vi "v4.1.vi"() -> ()   [LabVIEW 2018]
uses:
  <vilib>/DAQmx/read.llb/DAQmx Read (Analog 1D DBL NChan 1Samp).vi
  <extravilib>/ChannelInstances/High Speed Stream-c(a[.](c(dbl,dbl,dbl,dbl)),stamp,a[.](dbl),c(dbl,dbl,dbl,dbl,dbl,dbl,dbl))/_Read For Replicate.vi
  <extravilib>/ChannelInstances/High Speed Stream-c(a[.](c(dbl,dbl,dbl,dbl)),stamp,a[.](dbl),c(dbl,dbl,dbl,dbl,dbl,dbl,dbl))/Instantiate.vi
  <extravilib>/ChannelInstances/High Speed Stream-c(a[.](c(dbl,dbl,dbl,dbl)),stamp,a[.](dbl),c(dbl,dbl,dbl,dbl,dbl,dbl,dbl))/)Channel.vi
  <extravilib>/ChannelInstances/High Speed Stream-c(a[.](c(dbl,dbl,dbl,dbl)),stamp,a[.](dbl),c(dbl,dbl,dbl,dbl,dbl,dbl,dbl))/Abort Signal/Init Signal.vi
  <vilib>/Utility/file.llb/Write Delimited Spreadsheet (string).vi
  <vilib>/DAQmx/create/channels.llb/DAQmx Create Channel (AI-Temperature-Thermocouple).vi
  <vilib>/DAQmx/configure/timing.llb/DAQmx Timing (Sample Clock).vi
  <vilib>/DAQmx/miscellaneous.llb/DAQmx Fill In Error Info.vi
  <extravilib>/ChannelInstances/High Speed Stream-c(a[.](c(dbl,dbl,dbl,dbl)),stamp,a[.](dbl),c(dbl,dbl,dbl,dbl,dbl,dbl,dbl)).lvlib
  <resource>/objmgr/daqmx.rc
panel:
  out "Actual Sample Rate":dbl
  out "Export Timestamp":timestamp format="%<%H:%M:%S>T"
  out "Rig Temperatures":T1
  out "Flowrate Data":T2(array[cluster])
  out "UI Timestamp":timestamp format="%<%X\n%x>T"
  out "DAQ Timestamp":timestamp format="%<%H:%M:%S>T"
  in  "file path (dialog if empty)":path
  out "Enum":T3(ring)
  in  "Start Recording?":bool
  in  "Stop Recording?":bool
  in  "Flowrate Control":dbl
  out "Status":T4(ring)
  in  "OK Button":bool
  in  "DAQ Properties":cluster{"Sample Rate [Hz]":dbl}={"Sample Rate [Hz]"=1.0} {"Sample Rate [Hz]" min=0.1 max=10000.0 step=0.1}
  # "Line Data [ °C]"
  # "Rig Temperatures [ °C]"
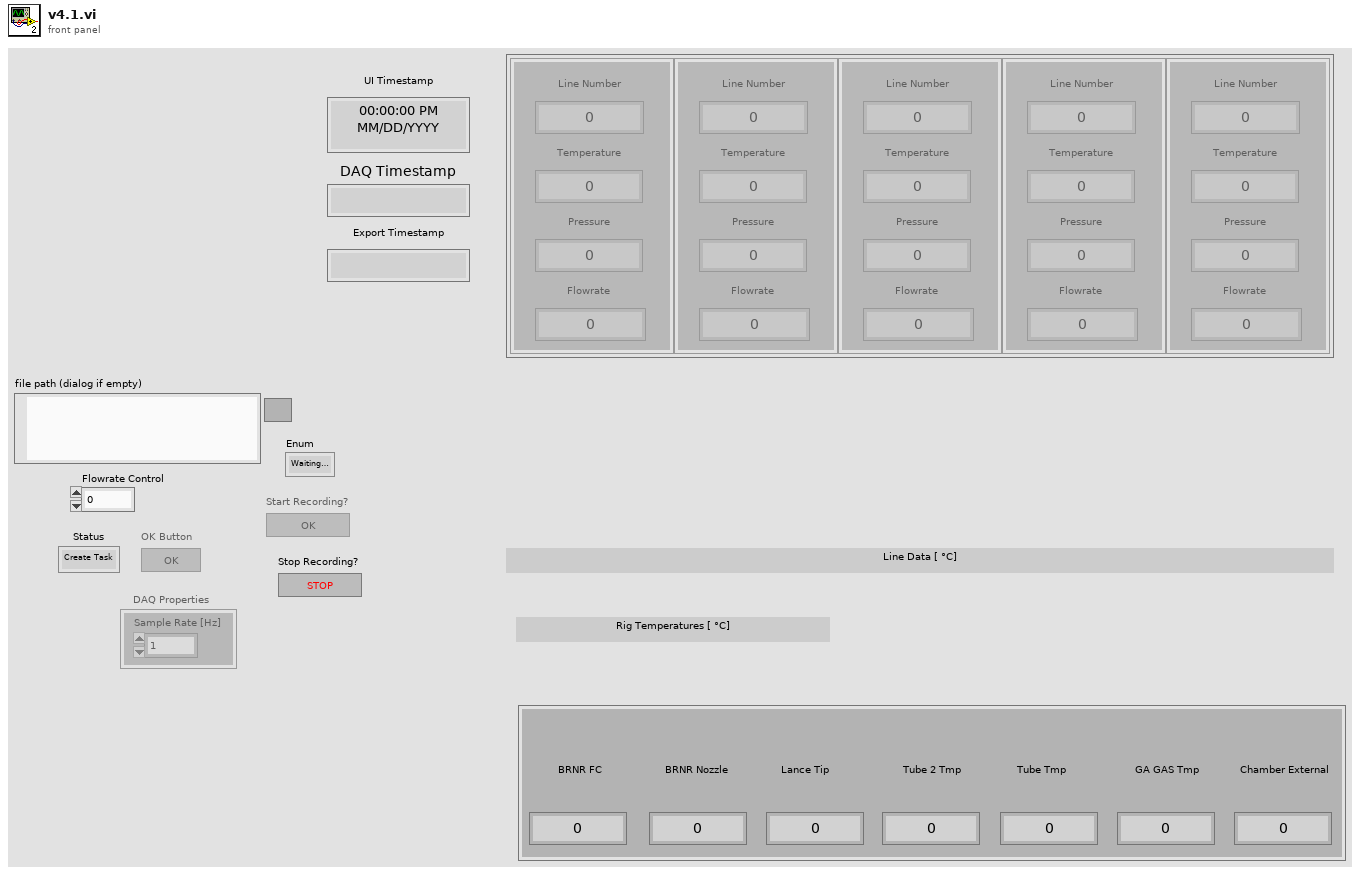
[diagram p1: front panel]
types:
  T1 = cluster{"BRNR FC":dbl, "BRNR Nozzle":dbl, "Lance Tip":dbl, "Tube 2 Tmp":dbl, "Tube Tmp":dbl, "GA GAS Tmp":dbl, "Chamber External":dbl}
  T2 = cluster{"Line Number":dbl, "Temperature":dbl, "Pressure":dbl, "Flowrate":dbl}[]
  T3 = enum16{"Waiting to record", "Creating Spreadsheet", "Recording", "Finished Recording"}
  T4 = enum16{"Create Task", "Change Settings", "Check Settings", "Read Data", "End Task"}
  T5 = enum8{"Enabled", "Disabled", "Disabled and Grayed Out"}
  T6 = cluster{"Flowrate Data":cluster{"Line Number":dbl, "Temperature":dbl, "Pressure":dbl, "Flowrate":dbl}[], "Current Time":timestamp, "DAQmx Data":dbl[], "Rig Temperatures":cluster{"BRNR FC":dbl, "BRNR Nozzle":dbl, "Lance Tip":dbl, "Tube 2 Tmp":dbl, "Tube Tmp":dbl, "GA GAS Tmp":dbl, "Chamber External Temp":dbl}}
  T7 = cluster{"BRNR FC":dbl, "BRNR Nozzle":dbl, "Lance Tip":dbl, "Tube 2 Tmp":dbl, "Tube Tmp":dbl, "GA GAS Tmp":dbl, "Chamber External Temp":dbl}
  T8 = typedef "High Speed Stream-c(a[.](c(dbl,dbl,dbl,dbl)),stamp,a[.](dbl),c(dbl,dbl,dbl,dbl,dbl,dbl,dbl)).lvlib/)Channel.ctl" = refnum<queue>
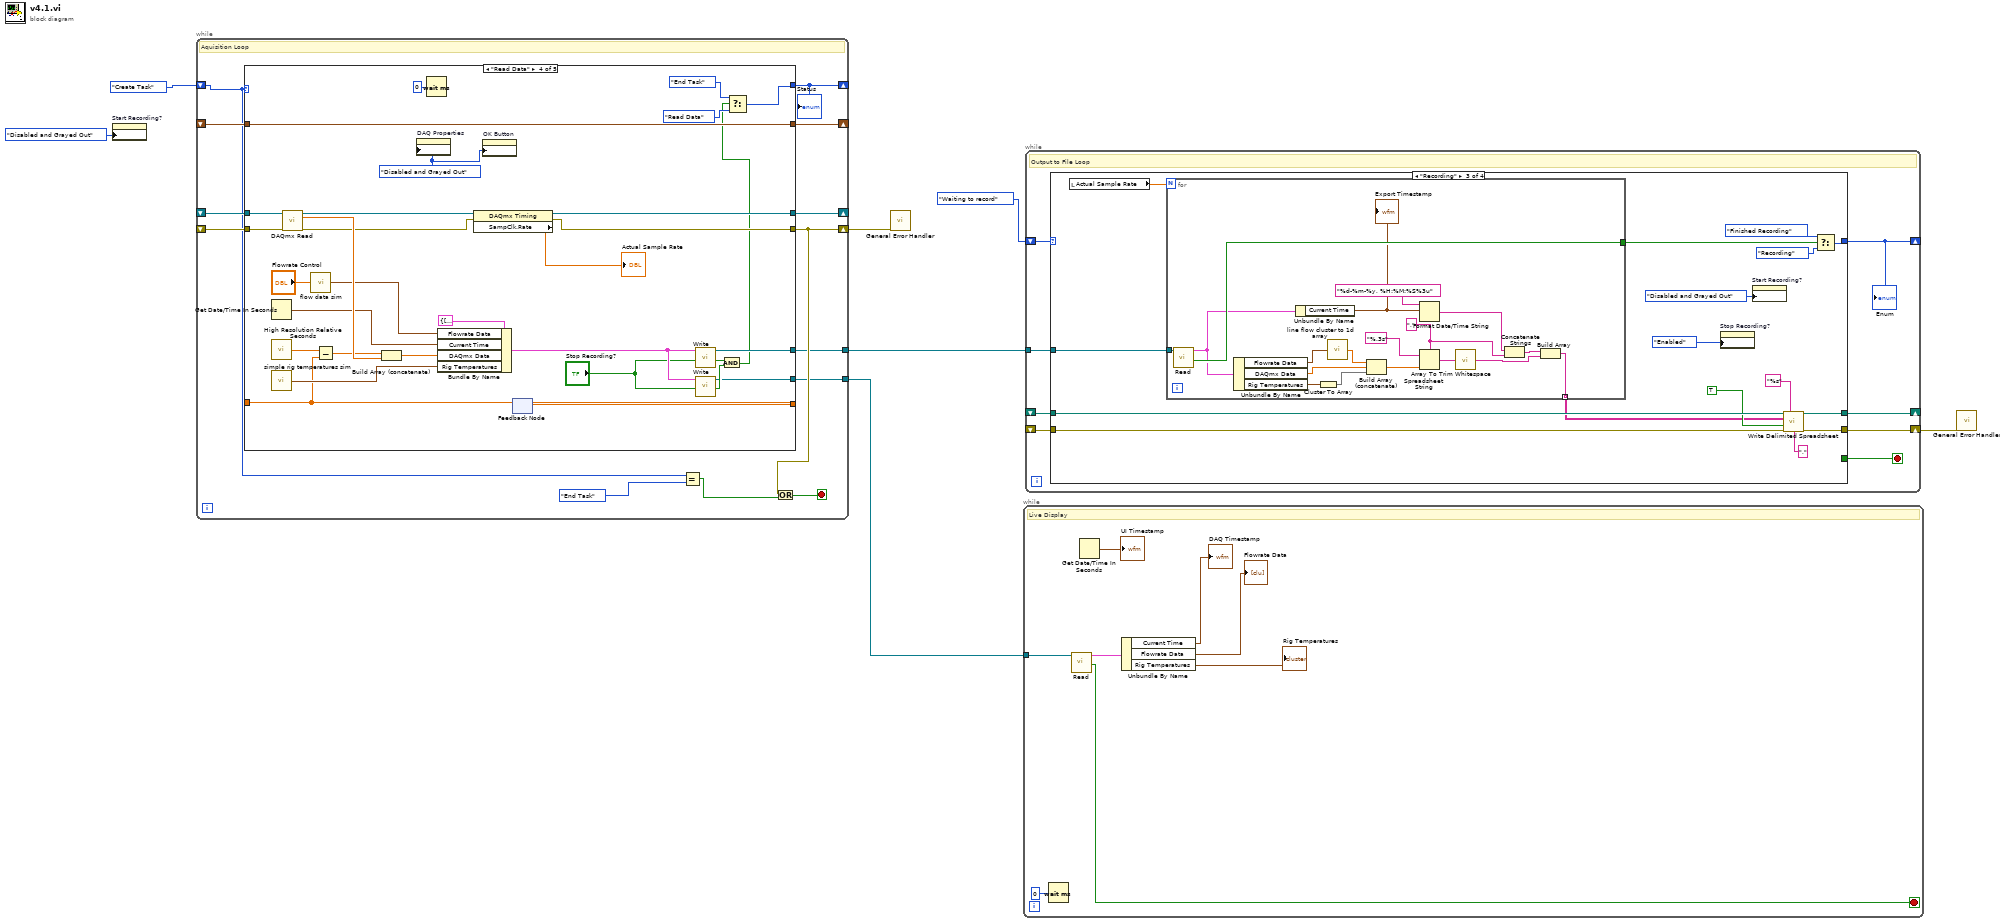
[diagram p0: block diagram]
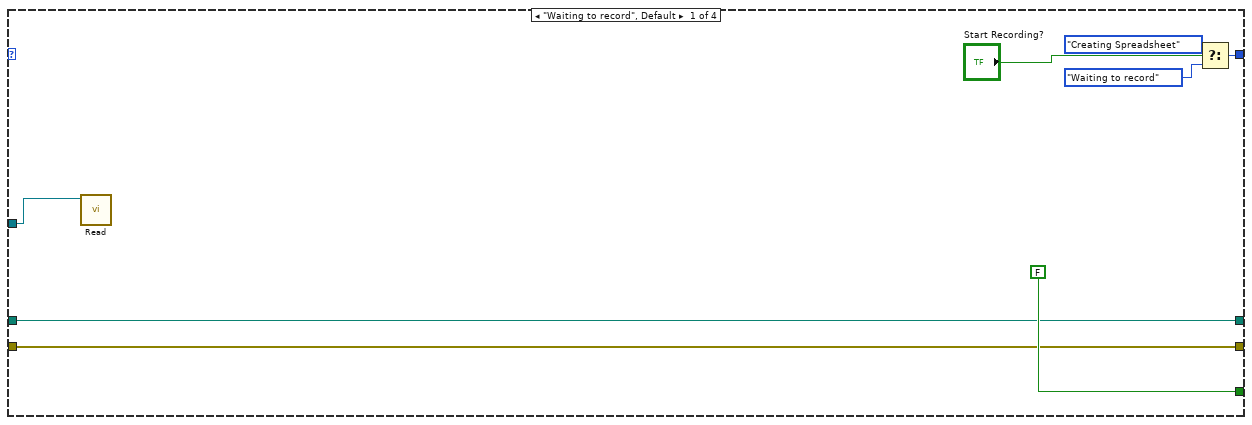
[diagram p2: hidden frame]
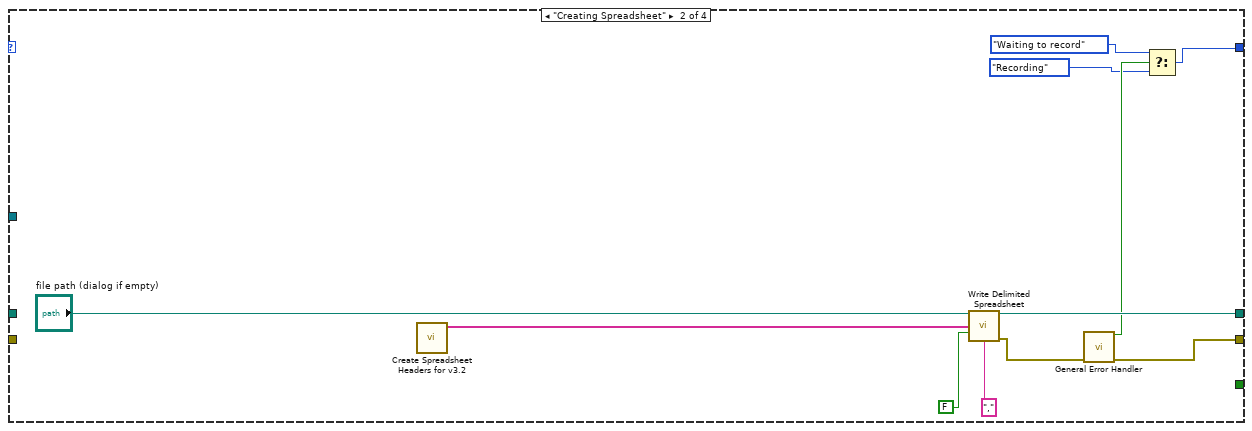
[diagram p3: hidden frame]
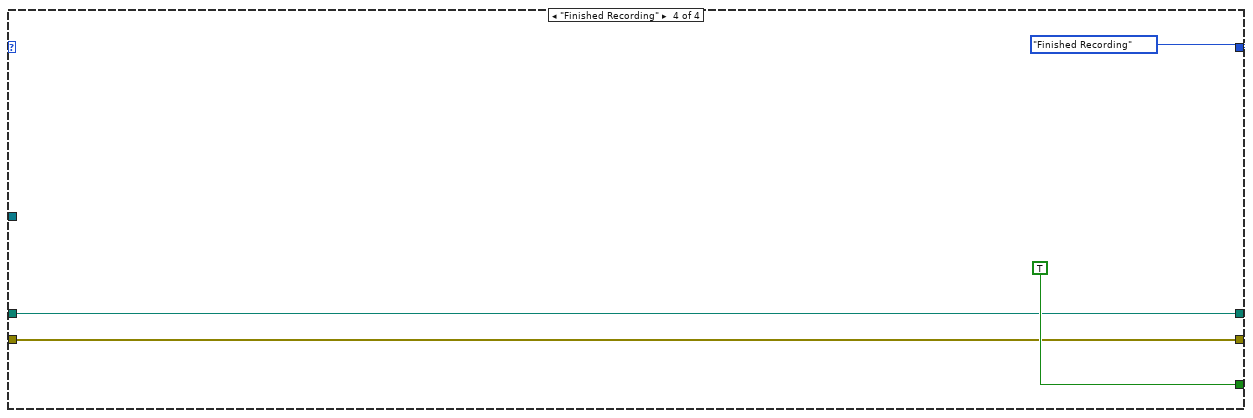
[diagram p4: hidden frame]
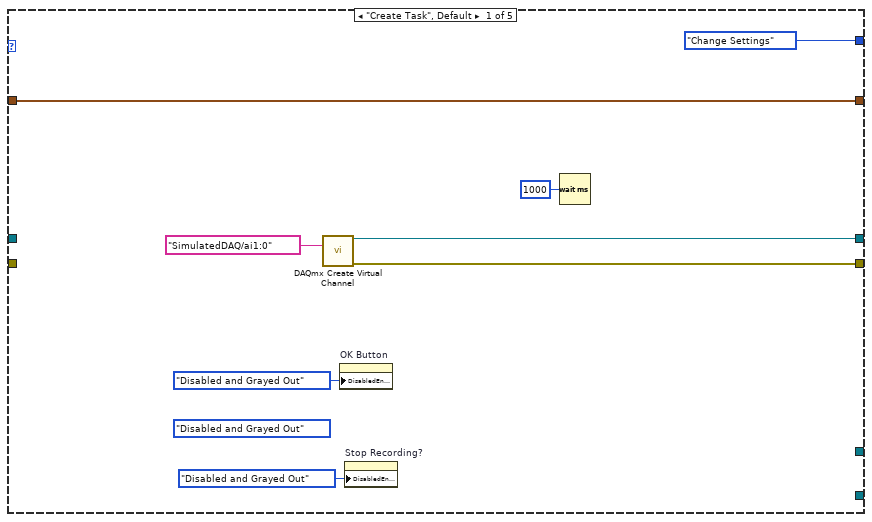
[diagram p5: hidden frame]
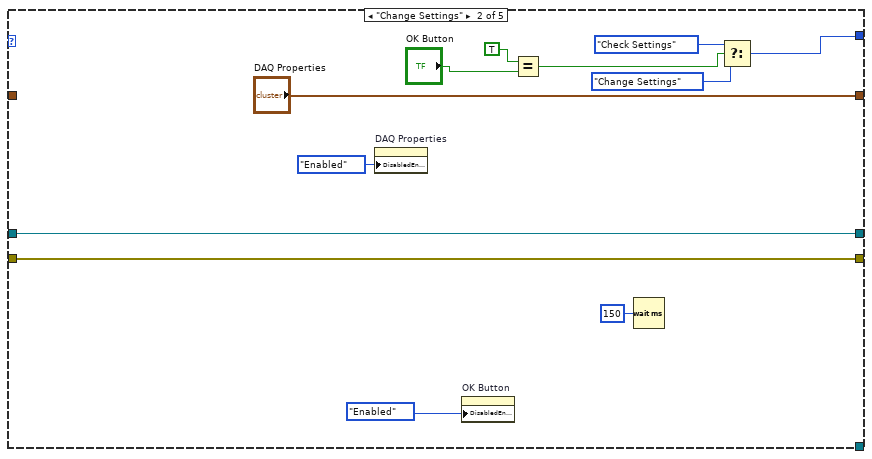
[diagram p6: hidden frame]
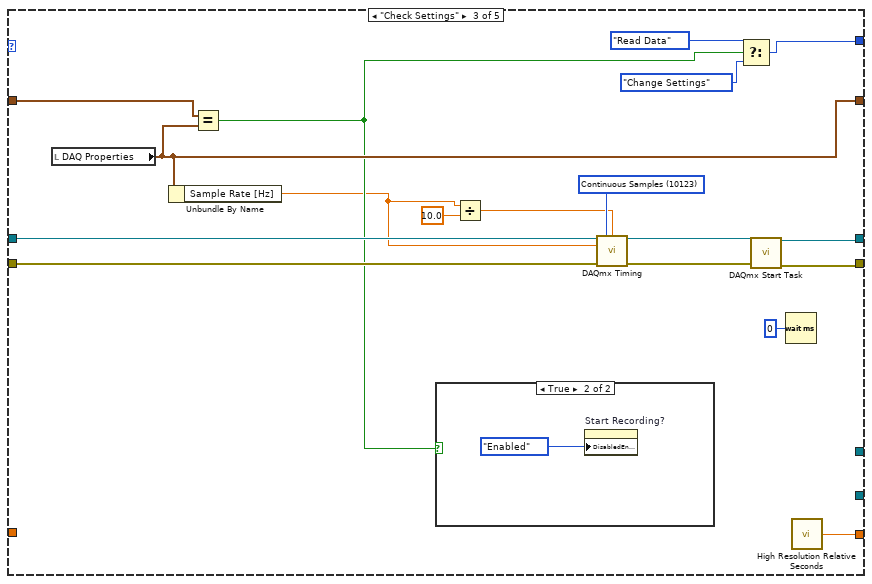
[diagram p7: hidden frame]
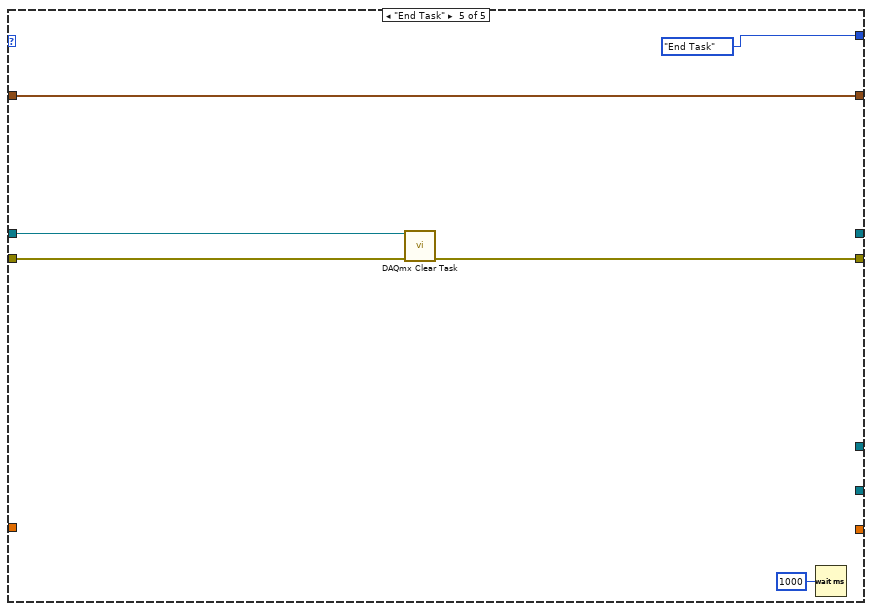
[diagram p9: hidden frame]
diagram:
  n1 = property on="Start Recording?" class="Bool"("DisabledEnum"=T5."Disabled and Grayed Out" ("Disabled")) -> ()  [unwired: 2 in, 2 out]
  n2 = while {
    shift-right: [w17] -> _
    shift-left: T4."Create Task" -> [w13]
    shift-right: [w22] -> _
    shift-left: _ -> [w20]
    shift-right: [w16] -> w3
    shift-left: _ -> [w19]
    shift-right: [w21] -> _
    shift-left: _ -> [w18]
    tunnel: [w11] -> w5
    tunnel: [w10] -> w1
    stop <- w12 stop-if-true
    # "Aquisition Loop"
    n3 = feedback #1() -> (w8:dbl)  [unwired: 1 in]
    n4 = case shown="\"Read Data\"" w13 {
      tunnel: [w30 w42 w50 w70 _] -> w22
      tunnel: [w29 w41 w49 w71 w97] -> w16
      tunnel: [T4."Change Settings" w35 w56 w87 T4."End Task"] -> w17
      tunnel: [w26 "DAQ Properties" w53 w89 w96] -> w21
      tunnel: w20 -> [_ w42 w55 w91 w94]
      tunnel: w19 -> [_ w41 w54 w90 w93]
      tunnel: w18 -> [w26 _ w60 w89 w96]
      tunnel: [_ _ _ w78 _] -> w11
      tunnel: [_ _ _ w67 _] -> w10
      tunnel: [_ _ w43 w62 _] -> w9
      tunnel: w8 -> [_ _ _ w62 _]
      frame "Create Task", Default {
        (unwired) T5."Disabled and Grayed Out" ("Disabled")
        n5 = call-poly <vilib>:"DAQmx Create Virtual Channel.vi"("physical channels"=tag "SimulatedDAQ/ai1:0") -> ("task out"=w30:refnum<k21>, "error out"=w29:errorcluster)  [unwired: 13 in]
        n6 = property on="OK Button" class="Bool"("DisabledEnum"=T5."Disabled and Grayed Out" ("Disabled")) -> ()  [unwired: 2 in, 2 out]
        n7 = property on="Stop Recording?" class="Bool"("DisabledEnum"=T5."Disabled and Grayed Out" ("Disabled")) -> ()  [unwired: 2 in, 2 out]
        n8 = Wait (ms)(milliseconds to wait=u32 1000) -> ()  [unwired: 1 out]
      }
      frame "Change Settings" {
        n9 = property on="DAQ Properties" class="Clust (strict)"("DisabledEnum"=T5."Enabled" ("Disabled")) -> ()  [unwired: 2 in, 2 out]
        n10 = property on="OK Button" class="Bool"("DisabledEnum"=T5."Enabled" ("Disabled")) -> ()  [unwired: 2 in, 2 out]
        n11 = Equal?(x=TRUE, y="OK Button") -> (x = y?=w37:bool)
        n12 = Wait (ms)(milliseconds to wait=u32 150) -> ()  [unwired: 1 out]
        n13 = Select(t=T4."Check Settings", s=w37, f=T4."Change Settings") -> (s? t:f=w35:T4)
      }
      frame "Check Settings" {
        w48 = 10123 items=["Finite Samples"=10178, "Continuous Samples"=10123, "Hardware Timed Single Point"=12522] ("sample mode")
        n14 = local read "DAQ Properties"() -> (w53:cluster{"Sample Rate [Hz]":dbl})
        n15 = Unbundle By Name(w53) -> ("Sample Rate [Hz]"=w45:dbl)
        n16 = Equal?(x=w60, y=w53) -> (x = y?=w47:bool)
        n17 = case shown="True" w47 {
          frame False {
          }
          frame True {
            n18 = property on="Start Recording?" class="Bool"("DisabledEnum"=T5."Enabled" ("Disabled")) -> ()  [unwired: 2 in, 2 out]
          }
        }
        n19 = Divide(x=w45, y=10.0) -> (x/y=w44:dbl)
        n20 = call-poly <vilib>:"DAQmx Timing.vi"("task/channels in"=w55, "sample mode"=w48, "samples per channel"=w44, "rate"=w45, "error in"=w54) -> ("task out"=w52:refnum<k21>, "error out"=w51:errorcluster)  [unwired: 9 in]
        n21 = Select(t=T4."Read Data", s=w47, f=T4."Change Settings") -> (s? t:f=w56:T4)
        n22 = call <vilib>:"DAQmx Start Task.vi"("task/channels in"=w52, "error in"=w51) -> ("task out"=w50:refnum<k21>, "error out"=w49:errorcluster)  [unwired: 12 in]
        n23 = Wait (ms)(milliseconds to wait=u32 0) -> ()  [unwired: 1 out]
        n24 = call <vilib>:"High Resolution Relative Seconds.vi"() -> ("relative seconds"=w43:dbl)
      }
      frame "Read Data" {
        w77 = T5."Disabled and Grayed Out" ("Disabled")
        n25 = Get Date/Time In Seconds() -> (seconds since 1Jan1904=w81:timestamp)
        n26 = call <vilib>:"High Resolution Relative Seconds.vi"() -> ("relative seconds"=w66:dbl)
        n27 = call "simple rig temperatures sim.vi"() -> ("Rig Temperatures"=w79:T7)
        n28 = call-poly <vilib>:"DAQmx Read.vi"("task/channels in"=w91, "error in"=w90) -> ("task out"=w72:refnum<k21>, "data"=w84:dbl[], "error out"=w69:errorcluster)  [unwired: 11 in]
        n29 = call "flow data sim.vi"("Offset"="Flowrate Control") -> ("Flowrate Data"=w80:T2)
        n30 = Subtract(x=w66, y=w62) -> (x-y=w63:dbl)
        n31 = Build Array (concatenate)(w63, w84) -> (w64:dbl[])
        n32 = property on="DAQ Properties" class="Clust (strict)"("DisabledEnum"=w77) -> ()  [unwired: 2 in, 2 out]
        n33 = Wait (ms)(milliseconds to wait=u32 0) -> ()  [unwired: 1 out]
        n34 = Bundle By Name(cluster=T6 {"Flowrate Data"=[{"Line Number"=1.0, "Temperature"=17.480721541683437, "Pressure"=24.0, "Flowrate"=0.0}, {"Line Number"=2.0, "Temperature"=21.850901927104296, "Pressure"=30.0, "Flowrate"=0.0}, {"Line Number"=3.0, "Temperature"=26.221082312525155, "Pressure"=36.0, "Flowrate"=0.0}, {"Line Number"=4.0, "Temperature"=30.591262697946018, "Pressure"=42.00000000000001, "Flowrate"=0.0}, {"Line Number"=5.0, "Temperature"=34.96144308336687, "Pressure"=48.0, "Flowrate"=0.0}], "Current Time"=timestamp(0 s since 1904-01-01), "DAQmx Data"=[], "Rig Temperatures"={"BRNR FC"=0.0, "BRNR Nozzle"=0.0, "Lance Tip"=0.0, "Tube 2 Tmp"=0.0, "Tube Tmp"=0.0, "GA GAS Tmp"=0.0, "Chamber External Temp"=0.0}}, "Flowrate Data"=w80, "Current Time"=w81, "DAQmx Data"=w64, "Rig Temperatures"=w79) -> (w76:T6)
        n35 = property class="DAQmx Timing"(reference=w72, error in=w69) -> (reference out=w70:refnum<k21>, error out=w71:errorcluster, "SampClk.Rate"=→"Actual Sample Rate":dbl)
        n36 = property on="OK Button" class="Bool"("DisabledEnum"=w77) -> ()  [unwired: 2 in, 2 out]
        n37 = call <extravilib>:"Write.vi"("last element? (F)"="Stop Recording?", "element"=w76) -> ("done?"=w74:bool, "channel"=w78:T8)  [unwired: 7 in, 1 out]
        n38 = call <extravilib>:"Write.vi"("last element? (F)"="Stop Recording?", "element"=w76) -> ("done?"=w73:bool, "channel"=w67:T8)  [unwired: 7 in, 1 out]
        n39 = And(x=w74, y=w73) -> (x .and. y?=w65:bool)
        n40 = Select(t=T4."End Task", s=w65, f=T4."Read Data") -> (s? t:f=w87:T4)
      }
      frame "End Task" {
        n41 = call <vilib>:"DAQmx Clear Task.vi"("task in"=w94, "error in"=w93) -> ("error out"=w97:errorcluster)  [unwired: 13 in]
        n42 = Wait (ms)(milliseconds to wait=u32 1000) -> ()  [unwired: 1 out]
      }
    }
    "Status" <- w17
    n43 = feedback-in #1(w9) -> ()
    n44 = Equal?(x=w13, y=T4."End Task") -> (x = y?=w14:bool)
    n45 = Or(x=w16, y=w14) -> (x .or. y?=w12:bool)
  }
  n46 = call <vilib>:"General Error Handler.vi"("error in (no error)"=w3) -> ()  [unwired: 10 in, 5 out]
  n47 = while {
    tunnel: w1 -> [w98]
    stop <- w105 stop-if-true
    # "Live Display"
    n48 = Wait (ms)(milliseconds to wait=u32 0) -> ()  [unwired: 1 out]
    n49 = call <extravilib>:"Read.vi"("channel"=w98) -> ("done?"=w105:bool, "element"=w103:T6)  [unwired: 6 in, 3 out]
    n50 = Get Date/Time In Seconds() -> (seconds since 1Jan1904=→"UI Timestamp":timestamp)
    n51 = Unbundle By Name(w103) -> ("Current Time"=→"DAQ Timestamp":timestamp, "Flowrate Data"=→"Flowrate Data":T2, "Rig Temperatures"=→"Rig Temperatures":T7)
  }
  n52 = while {
    shift-right: [w113] -> _
    shift-left: T3."Waiting to record" -> [w112]
    tunnel: w5 -> [w110]
    shift-right: [w108] -> _
    shift-left: _ -> [w109]
    shift-right: [w107] -> w4
    shift-left: _ -> [w106]
    stop <- w111 stop-if-true
    # "Output to File Loop"
    n53 = case shown="\"Recording\"" w112 {
      tunnel: [w118 w124 w147 T3."Finished Recording"] -> w113
      tunnel: [FALSE _ _ TRUE] -> w111
      tunnel: w110 -> [w114 _ w144 _]
      tunnel: w109 -> [w116 _ w141 w168]
      tunnel: [w116 w132 w142 w168] -> w108
      tunnel: [w115 w126 w136 w167] -> w107
      tunnel: w106 -> [w115 _ w139 w167]
      frame "Waiting to record", Default {
        n54 = call <extravilib>:"Read.vi"("channel"=w114) -> ()  [unwired: 6 in, 5 out]
        n55 = Select(t=T3."Creating Spreadsheet", s="Start Recording?", f=T3."Waiting to record") -> (s? t:f=w118:T3)
      }
      frame "Creating Spreadsheet" {
        n56 = call "Create Spreadsheet Headers for v3.2.vi"() -> ("Array"=w131:string[])  [unwired: 11 in]
        n57 = call-poly <vilib>:"Write Delimited Spreadsheet.vi"("file path (dialog if empty)"="file path (dialog if empty)", "1D data"=w131, "append to file? (new file:F)"=FALSE, "delimiter (\\t)"="," ("delimiter (\\t)")) -> ("new file path (Not A Path if cancelled)"=w132:path, "error out"=w127:errorcluster)  [unwired: 10 in]
        n58 = call <vilib>:"General Error Handler.vi"("error in (no error)"=w127) -> ("error?"=w125:bool, "error out"=w126:errorcluster)  [unwired: 10 in, 3 out]
        n59 = Select(t=T3."Waiting to record", s=w125, f=T3."Recording") -> (s? t:f=w124:T3)
      }
      frame "Recording" {
        n60 = local read "Actual Sample Rate"() -> (w133:dbl)
        n61 = for {
          N: w133 -> [_]
          tunnel: w144 -> [w165]
          tunnel: [w164] -> w143
          tunnel: [w149] -> w134 mode=indexing
          w154 = "," ("delimiter (Tab)")
          n62 = call <extravilib>:"Read.vi"("channel"=w165) -> ("done?"=w164:bool, "element"=w162:T6)  [unwired: 6 in, 3 out]
          n63 = Unbundle By Name(w162) -> ("Flowrate Data"=w163:T2, "DAQmx Data"=w160:dbl[], "Rig Temperatures"=w166:T7)
          n64 = Unbundle By Name(w162) -> ("Current Time"=w155:timestamp)
          "Export Timestamp" <- w155
          n65 = Cluster To Array(cluster=w166) -> (array=w161:dbl[])
          n66 = call "line flow cluster to 1d array.vi"("Flowrate Data"=w163) -> ("Array"=w159:dbl[])
          n67 = Build Array (concatenate)(w159, w160, w161) -> (w152:dbl[])
          n68 = Format Date/Time String(time format string (%c)="%d-%m-%y, %H:%M:%S%3u", seconds (now)=w155) -> (date/time string=w153:string)  [unwired: 1 in]
          n69 = Array To Spreadsheet String(delimiter (Tab)=w154, array=w152, 3:"%.3s" ("format string")) -> (spreadsheet string=w158:string)
          n70 = call <vilib>:"Trim Whitespace.vi"("string"=w158) -> ("trimmed string"=w150:string)  [unwired: 1 in]
          n71 = Concatenate Strings(w153, w154) -> (w151:string)
          n72 = Build Array(w151, w150) -> (w149:string[])
        }
        n73 = property on="Stop Recording?" class="Bool"("DisabledEnum"=T5."Enabled" ("Disabled")) -> ()  [unwired: 2 in, 2 out]
        n74 = property on="Start Recording?" class="Bool"("DisabledEnum"=T5."Disabled and Grayed Out" ("Disabled")) -> ()  [unwired: 2 in, 2 out]
        n75 = call-poly <vilib>:"Write Delimited Spreadsheet.vi"("file path (dialog if empty)"=w141, "format (%s)"="%s", "2D data"=w134, "append to file? (new file:F)"=TRUE, "error in (no error)"=w139, "delimiter (\\t)"="," ("delimiter (\\t)")) -> ("new file path (Not A Path if cancelled)"=w142:path, "error out"=w136:errorcluster)  [unwired: 8 in]
        n76 = Select(t=T3."Finished Recording", s=w143, f=T3."Recording") -> (s? t:f=w147:T3)
      }
      frame "Finished Recording" {
      }
    }
    "Enum" <- w113
  }
  n77 = call <vilib>:"General Error Handler.vi"("error in (no error)"=w4) -> ()  [unwired: 10 in, 5 out]
